vi "options.vi"(8 "Error In":errorcluster, 11 "QFileDialog In":refnum<class "QFileDialog.lvclass">) -> (0 "Error Out":errorcluster, 2 "Value":T1=1 items=["ShowDirsOnly"=1, "DontResolveSymlinks"=2, "DontConfirmOverwrite"=4, "DontUseSheet"=8, "DontUseNativeDialog"=16, "ReadOnly"=32, "HideNameFilterDetails"=64, "DontUseCustomDirectoryIcons"=128], 3 "QFileDialog Out":refnum<class "QFileDialog.lvclass">)   [LabVIEW 2014, in "QFileDialog.lvclass"]
doc: "LabVIEW-specific documentation is not yet available. See <b>https://doc.qt.io/qt-5/qfiledialog.html#options</b>"
uses:
  QFileDialog.lvclass
  Option.ctl
  LQ Core/LQIdentity/LQIdentity.lvclass/LQIdentity.ctl
  LQ Core/LQ Core.lvlib
  LQ Core/LQIdentity/LQIdentity.lvclass
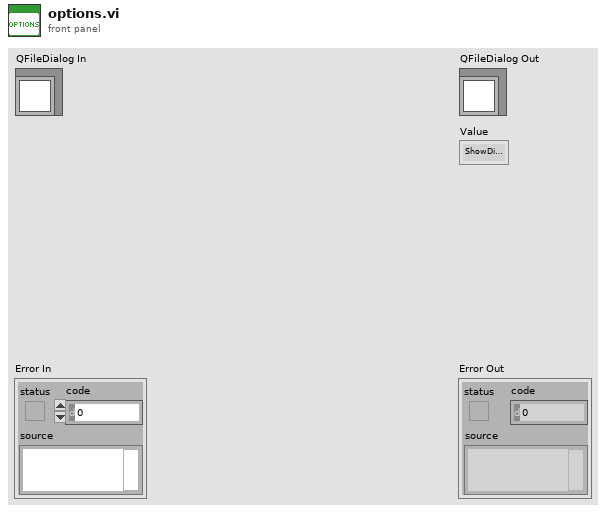
[diagram p1: front panel]
types:
  T1 = typedef "QFileDialog.lvclass/Option.ctl" = i32
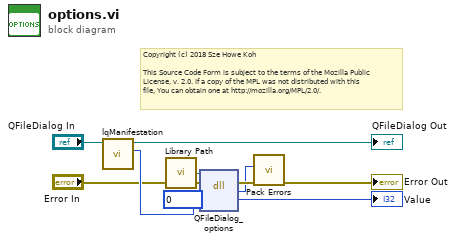
[diagram p0: block diagram]
diagram:
  w7 = T1 0 items=["ShowDirsOnly"=1, "DontResolveSymlinks"=2, "DontConfirmOverwrite"=4, "DontUseSheet"=8, "DontUseNativeDialog"=16, "ReadOnly"=32, "HideNameFilterDetails"=64, "DontUseCustomDirectoryIcons"=128] ("retVal")
  # "Copyright (c) 2018 Sze Howe Koh\n\nThis Source Code Form is subject to the terms of the Mozilla Public\nLicense, v. 2.0. If a copy of the MPL was not distributed with this\nfile, You can obtain one at http://mozilla.org/MPL/2.0/."
  n1 = call "lqManifestation.vi"("LQIdentity in"="QFileDialog In") -> ("Manifestation"=w5:u64, "LQIdentity out"=→"QFileDialog Out":refnum<class "QFileDialog.lvclass">)  [unwired: 9 in]
  n2 = call "Library Path.vi"() -> ("Library Path"=w6:path)
  n3 = dll-call lib="?" fn="QFileDialog_options"(path in=w6, error in="Error In", "_retVal"=w7, "_instance"=w5) -> (error out=w3:errorcluster, w1:i32, "_retVal"=→"Value":i32)  [unwired: 2 in, 1 out]
  n4 = call "Pack Errors.vi"("Error In"=w3, "Error Code"=w1) -> ("Error Out"=→"Error Out":errorcluster)  [unwired: 9 in]
